vi "Reset WT210 Integrator.vi"(8 "error in (no error)":errorcluster, 11 "VISA resource name":refnum<visa-resource-name>) -> (0 "error out":errorcluster, 3 "VISA resource name out":refnum<visa-resource-name>)   [LabVIEW 2018]
uses:
  Yokogawa WT200 Series.lvlib
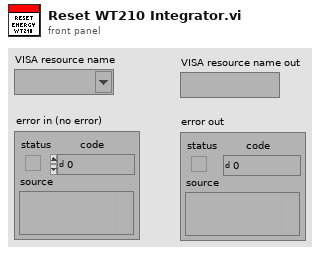
[diagram p1: front panel]
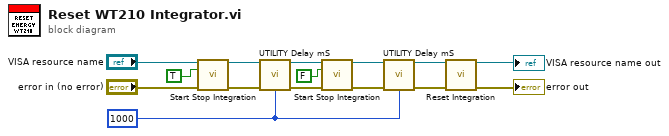
[diagram p0: block diagram]
diagram:
  w3 = u32 1000 ("milliseconds to wait")
  n1 = call "Start Stop Integration.vi"("VISA resource name"="VISA resource name", "Start/Stop (F: Stop)"=TRUE, "error in (no error)"="error in (no error)") -> ("VISA resource name out"=w8:refnum<visa-resource-name>, "error out"=w10:errorcluster)  [unwired: 11 in]
  n2 = call "UTILITY Delay mS.vi"("Error In"=w10, "milliseconds to wait"=w3) -> ("Error Out"=w11:errorcluster)  [unwired: 13 in]
  n3 = call "Start Stop Integration.vi"("VISA resource name"=w8, "Start/Stop (F: Stop)"=FALSE, "error in (no error)"=w11) -> ("VISA resource name out"=w9:refnum<visa-resource-name>, "error out"=w12:errorcluster)  [unwired: 11 in]
  n4 = call "UTILITY Delay mS.vi"("Error In"=w12, "milliseconds to wait"=w3) -> ("Error Out"=w13:errorcluster)  [unwired: 13 in]
  n5 = call "Reset Integration.vi"("VISA resource name"=w9, "error in (no error)"=w13) -> ("VISA resource name out"=→"VISA resource name out":refnum<visa-resource-name>, "error out"=→"error out":errorcluster)  [unwired: 12 in]
